vi "Load Background.vi"(7 "Group":string="Raw", 8 "error in (no error)":errorcluster, 9 "Channel":string="Avg Amplitude", 10 "Background":path, 11 "Ocean Optics Driver in":refnum<class "Ocean Optics Driver.lvclass">) -> (0 "error out":errorcluster, 3 "Ocean Optics Driver out":refnum<class "Ocean Optics Driver.lvclass">)   [LabVIEW 2016, in "Ocean Optics Driver.lvclass"]
uses:
  Ocean Optics Driver.lvclass
  Ocean Optics Driver.lvclass/Ocean Optics Driver.ctl
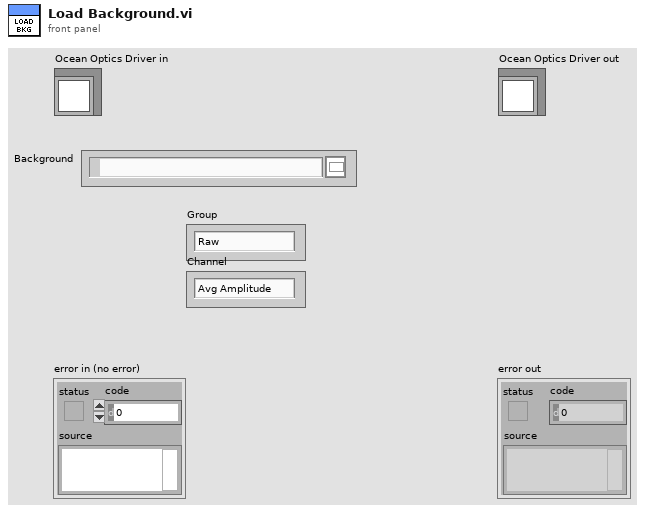
[diagram p1: front panel]
types:
  T1 = enum16{"open", "open or create", "create or replace", "create", "open (read-only)"}
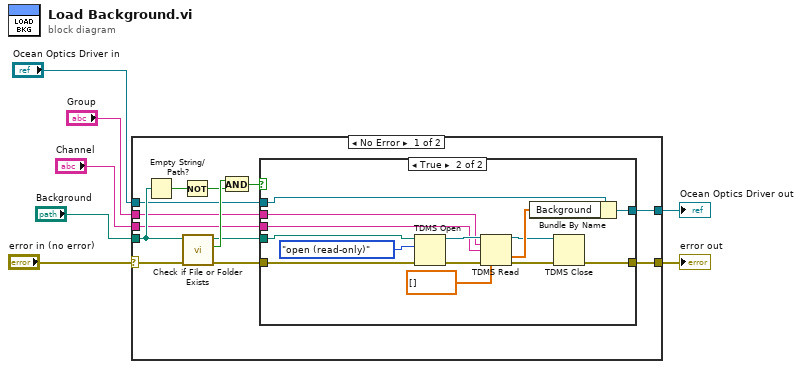
[diagram p0: block diagram]
diagram:
  n1 = case shown="No Error" "error in (no error)" {
    selector: "error in (no error)" -> [w14 w38]
    tunnel: [w8 w38] -> w6
    tunnel: [w9 w37] -> w4
    tunnel: "Ocean Optics Driver in" -> [w10 w37]
    tunnel: "Background" -> [w20 _]
    tunnel: "Group" -> [w12 _]
    tunnel: "Channel" -> [w11 _]
    frame No Error {
      n2 = Empty String/Path?(string/path=w20) -> (empty?=w19:bool)
      n3 = Not(x=w19) -> (.not. x?=w17:bool)
      n4 = call <vilib>:"Check if File or Folder Exists.vi"("error in (no error)"=w14, "path"=w20) -> ("error out"=w13:errorcluster, "file or folder exists?"=w18:bool, "dup path"=w15:path)  [unwired: 7 in]
      n5 = And(x=w18, y=w17) -> (x .and. y?=w16:bool)
      n6 = case shown="True" w16 {
        tunnel: w13 -> [w21 w36]
        tunnel: w15 -> [_ w34]
        tunnel: w12 -> [_ w31]
        tunnel: w11 -> [_ w29]
        tunnel: w10 -> [w22 w28]
        tunnel: [w22 w27] -> w9
        tunnel: [w21 w23] -> w8
        frame False {
        }
        frame True {
          n7 = TDMS Open(8:w36, 10:T1."open (read-only)" ("operation (0:open)"), 11:w34) -> (0:w32:errorcluster, 3:w33:refnum<k34>)  [unwired: 4 in]
          n8 = TDMS Read(0:w33, 5:w31, 7:w29, 11:w32, 12:dbl[] []) -> (4:w24:refnum<k34>, 10:w26:dbl[], 15:w25:errorcluster)  [unwired: 3 in, 3 out]
          n9 = Bundle By Name(cluster=w28, "Background"=w26) -> (w27:refnum<class "Ocean Optics Driver.lvclass">)
          n10 = TDMS Close(8:w25, 11:w24) -> (0:w23:errorcluster)  [unwired: 1 out]
        }
      }
    }
    frame Error {
    }
  }
  "error out" <- w6
  "Ocean Optics Driver out" <- w4
